vi "Configure Trace.vi"(8 "error in (no error)":errorcluster, 9 "Enable Trace Mode (T: Enable)":bool=TRUE, 10 "Trace (0: Channel 1)":u16(ring) items=["Channel 1", "Channel 2", "Channel 3", "Channel 4", "Memory 1", "Memory 2", "Memory 3", "Memory 4", "Function 1", "Function 2", "Function 3", "Function 4", "Function 5", "Function 6", "Function 7", "Function 8"], 11 "VISA resource name":refnum<visa-resource-name>) -> (0 "error out":errorcluster, 3 "VISA resource name out":refnum<visa-resource-name>)   [LabVIEW 2015, in "LeCroy Wave Series.lvlib"]
doc: "Specify whether you want the oscilloscope enabled to acquire data for the specified trace."
uses:
  <instrlib>/LeCroy Wave Series/LeCroy Wave Series.lvlib
panel:
  # "Enable\n\nDisable"
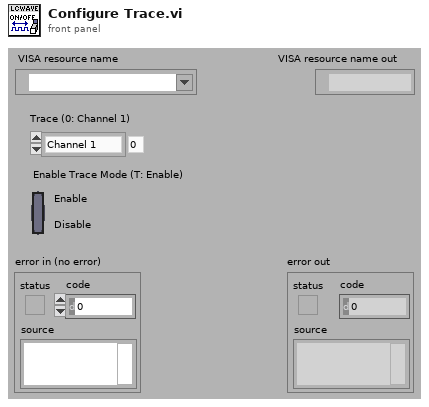
[diagram p1: front panel]
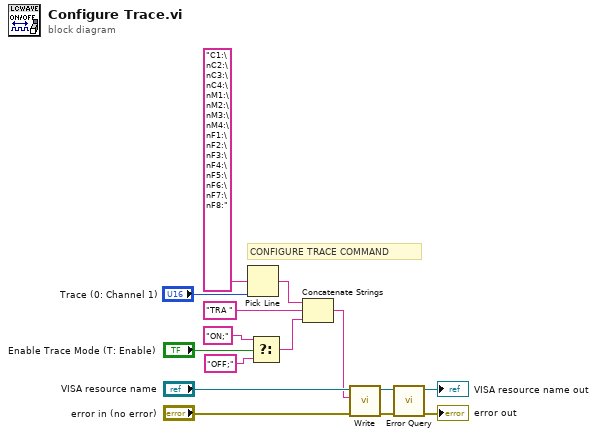
[diagram p0: block diagram]
diagram:
  # "CONFIGURE TRACE COMMAND"
  n1 = Pick Line(multi-line string="C1:\nC2:\nC3:\nC4:\nM1:\nM2:\nM3:\nM4:\nF1:\nF2:\nF3:\nF4:\nF5:\nF6:\nF7:\nF8:", line index="Trace (0: Channel 1)") -> (output string=w4:string)  [unwired: 1 in]
  n2 = Select(t="ON;", s="Enable Trace Mode (T: Enable)", f="OFF;") -> (s? t:f=w2:string)
  n3 = Concatenate Strings(w4, "TRA ", w2) -> (w1:string)
  n4 = call <instrlib>:"Write.vi"("error in (no error)"="error in (no error)", "Write Buffer"=w1, "VISA resource name"="VISA resource name") -> ("error out"=w10:errorcluster, "VISA resource name out"=w11:refnum<visa-resource-name>)  [unwired: 6 in, 1 out]
  n5 = call <instrlib>:"Error Query.vi"("error in (no error)"=w10, "VISA resource name"=w11) -> ("error out"=→"error out":errorcluster, "VISA resource name out"=→"VISA resource name out":refnum<visa-resource-name>)  [unwired: 6 in, 2 out]
